vi "Test Smoothing - ALL.vi"() -> ()   [LabVIEW 2013]
panel:
  in  "Mode":enum8{"Off", "Stby", "Hold", "Run"}(ring)=enum."Stby"
  out "PO2":dbl=18003.97265625
  out "System Status Out":bool
  out "Alt Eff correct":dbl=1449.1019287109375
  out "O2%-2":dbl=21.433300018310547
  out "O2%-1":dbl=21.433300018310547
  out "Waveform Chart":dbl(graph)
  in  "O2ppm 2":u32=209400
  in  "O2ppm":u32=209400
  in  "Random":bool
  in  "Boolean":bool
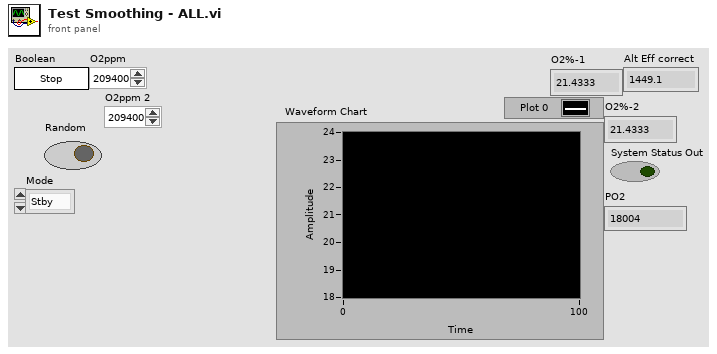
[diagram p1: front panel]
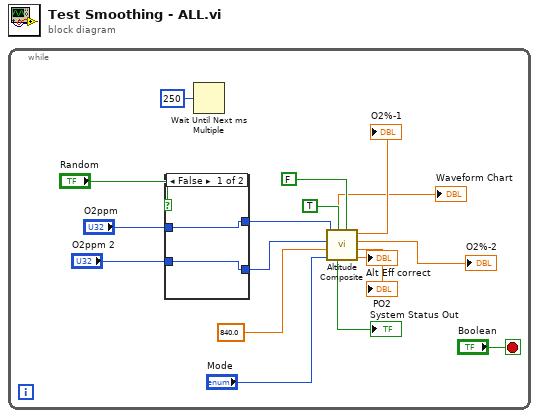
[diagram p0: block diagram]
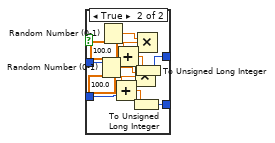
[diagram p2: hidden frame]
diagram:
  n1 = while {
    stop <- "Boolean" stop-if-true
    n2 = case shown="False" "Random" {
      tunnel: "O2ppm" -> [w19 w31]
      tunnel: [w19 w26] -> w11
      tunnel: "O2ppm 2" -> [w18 w21]
      tunnel: [w18 w20] -> w9
      frame False {
      }
      frame True {
        n3 = Random Number (0-1)() -> (number: 0 to 1=w22:dbl)
        n4 = Random Number (0-1)() -> (number: 0 to 1=w30:dbl)
        n5 = Multiply(x=w22, y=100.0) -> (x*y=w24:dbl)
        n6 = Add(x=w24, y=w21) -> (x+y=w25:dbl)
        n7 = To Unsigned Long Integer(number=w25) -> (unsigned 32bit integer=w20:u32)
        n8 = Multiply(x=w30, y=100.0) -> (x*y=w28:dbl)
        n9 = Add(x=w28, y=w31) -> (x+y=w27:dbl)
        n10 = To Unsigned Long Integer(number=w27) -> (unsigned 32bit integer=w26:u32)
      }
    }
    n11 = Wait Until Next ms Multiple(millisecond multiple=u32 250) -> ()  [unwired: 1 out]
    n12 = call "Altitude Composite.vi"("Feet OFF/ Meters ON"=FALSE, "West ON/Std OFF"=TRUE, "Mode"="Mode", "Pressure mBar"=840.0, "O2ppm-2"=w9, "O2ppm-1"=w11) -> ("PO2"=→"PO2":dbl, "Alt Eff correct"=→"Alt Eff correct":dbl, "O2%-2"=→"O2%-2":dbl, "O2%-1"=→"O2%-1":dbl, "System Status Out"=→"System Status Out":bool, "Mean O2%"=→"Waveform Chart":dbl)
  }
